vi "Setup.vi"(0 "Path in":refnum<class "Path.lvclass">, 11 "error in (no error)":errorcluster) -> (4 "Path out":refnum<class "Path.lvclass">, 15 "error out":errorcluster)   [LabVIEW 2023, in "RFCalAndFixtureCharact.Common.lvlib" / "Path.lvclass"]
uses:
  Path.lvclass
  Fixture/Public/RFFixtureCharact.Public.lvlib
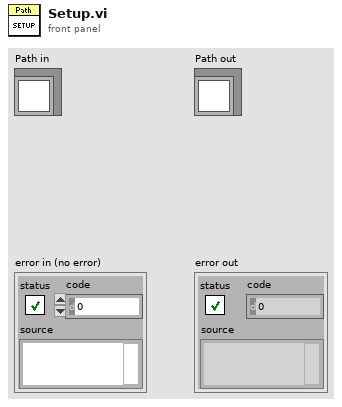
[diagram p1: front panel]
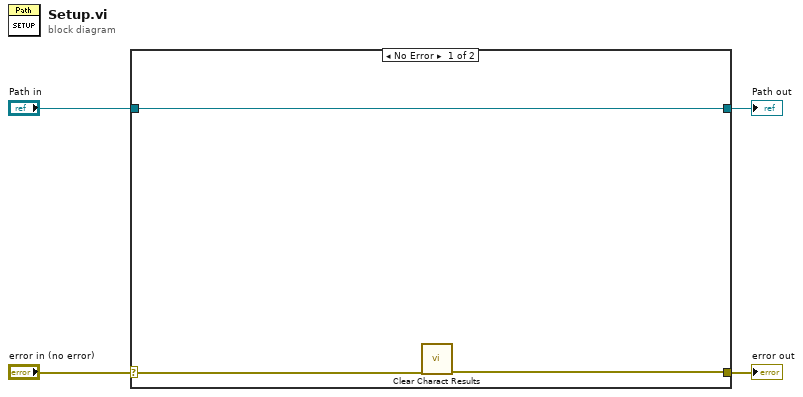
[diagram p0: block diagram]
diagram:
  n1 = case shown="No Error" "error in (no error)" {
    selector: "error in (no error)" -> [w6 w9]
    tunnel: [w5 w9] -> w3
    tunnel: [w7 w8] -> w1
    tunnel: "Path in" -> [w7 w8]
    frame No Error {
      n2 = call "Clear Charact Results.vi"("error in"=w6) -> ("error out"=w5:errorcluster)  [unwired: 14 in]
    }
    frame Error {
    }
  }
  "error out" <- w3
  "Path out" <- w1
